vi "Lab 1.vi"() -> ()   [LabVIEW 2014]
panel:
  out "Odd Number":bool
  out "Even Number":bool
  out "Number > 5?":bool
  out "Random Number Generated":dbl
  out "Fahrenheit (F)":dbl
  out "Celsius (C)":dbl
  in  "Volt (V)":dbl
  out "Celsius (C)":dbl(slide) scale=0.0..100.0
  in  "Fahrenheit (F)":dbl(slide) scale=0.0..100.0
  out "Fahrenheit (F)":dbl
  in  "Celsius (C)":dbl
  # "Converts Celsius to Fahrenheit"
  # "Converts Fahrenheit to Celsius"
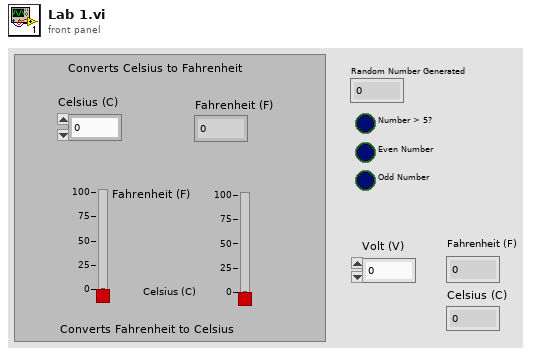
[diagram p1: front panel]
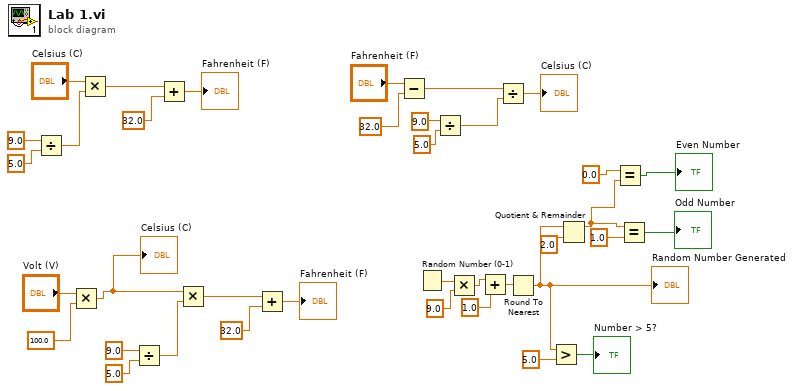
[diagram p0: block diagram]
diagram:
  n1 = Divide(x=9.0, y=5.0) -> (x/y=w33:dbl)
  n2 = Multiply(x="Volt (V)", y=100.0) -> (x*y=w15:dbl)
  "Celsius (C)" <- w15
  n3 = Multiply(x="Celsius (C)", y=w33) -> (x*y=w32:dbl)
  n4 = Divide(x=9.0, y=5.0) -> (x/y=w18:dbl)
  n5 = Add(x=w32, y=32.0) -> (x+y=→"Fahrenheit (F)":dbl)
  n6 = Multiply(x=w15, y=w18) -> (x*y=w17:dbl)
  n7 = Add(x=w17, y=32.0) -> (x+y=→"Fahrenheit (F)":dbl)
  n8 = Subtract(x="Fahrenheit (F)", y=32.0) -> (x-y=w28:dbl)
  n9 = Random Number (0-1)() -> (number: 0 to 1=w14:dbl)
  n10 = Divide(x=9.0, y=5.0) -> (x/y=w24:dbl)
  n11 = Multiply(x=w14, y=9.0 ("number (0 to 1)")) -> (x*y=w2:dbl)
  n12 = Add(x=w2, y=1.0) -> (x+y=w3:dbl)
  n13 = Divide(x=w28, y=w24) -> (x/y=→"Celsius (C)":dbl)
  n14 = Round To Nearest(number=w3) -> (nearest integer value=w5:dbl)
  "Random Number Generated" <- w5
  n15 = Greater?(x=w5, y=5.0) -> (0:→"Number > 5?":bool)
  n16 = Quotient & Remainder(x=w5, y=2.0) -> (x-y*floor(x/y)=w6:dbl)  [unwired: 1 out]
  n17 = Equal?(x=0.0, y=w6) -> (x = y?=→"Even Number":bool)
  n18 = Equal?(x=w6, y=1.0) -> (x = y?=→"Odd Number":bool)
